vi "GetCurrentSnapshot.vi"(8 "error in (no error)":errorcluster, 11 "Logger in":refnum<class "Logger.lvclass">) -> (0 "error out":errorcluster, 2 "Snapshot":T1={"globalThreshold"=enum."INFO", "appenders"=[]}, 3 "Logger out":refnum<class "Logger.lvclass">)   [LabVIEW 2026, in "Lumberjack.lvlib" / "Logger.lvclass"]
doc: "Reads the logger's current published Snapshot without consuming it.\nNon-destructively reads the shared Snapshot notifier and returns globalThreshold plus the appenders array (RegistryEntry {id, enqueuer}) the manager last posted; reflects the state as of the last register/unregister/threshold change. Returns the empty/default Snapshot when no logger resolves.\nLumberjack.lvlib, Logger.lvclass, public."
uses:
  Logger.lvclass
  TypeDefs/Snapshot.ctl
  TypeDefs/Severity.ctl
  <vilib>/ActorFramework/Message Enqueuer/Message Enqueuer.lvclass
  Logger.lvclass/Logger.ctl
  Lumberjack.lvlib
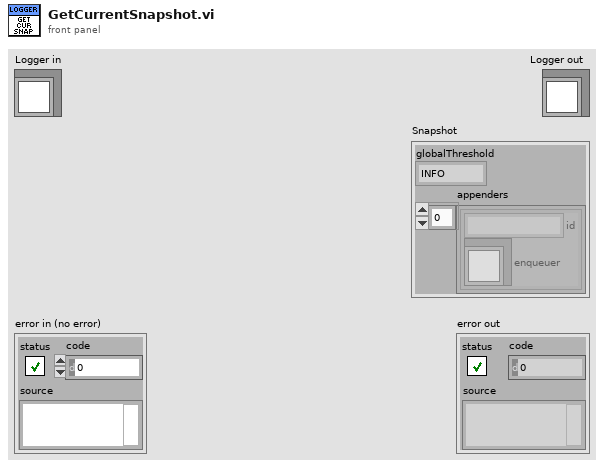
[diagram p1: front panel]
types:
  T1 = typedef "Lumberjack.lvlib/Snapshot.ctl" = cluster{"globalThreshold":T2, "appenders":cluster{"id":string, "enqueuer":refnum<class "Message Enqueuer.lvclass">}[]}
  T2 = typedef "Lumberjack.lvlib/Severity.ctl" = enum16{"OFF", "FATAL", "ERROR", "WARN", "INFO", "DEBUG", "TRACE", "ALL"}
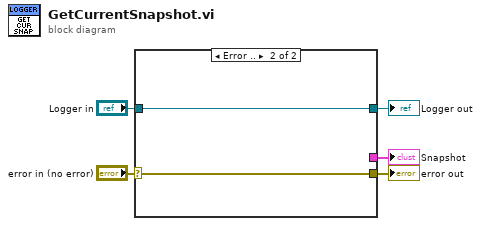
[diagram p0: block diagram]
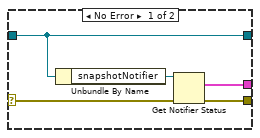
[diagram p2: hidden frame]
diagram:
  n1 = case shown="Error .." "error in (no error)" {
    selector: "error in (no error)" -> [w7 w12]
    tunnel: [w10 w12] -> w5
    tunnel: [w8 _] -> w4
    tunnel: "Logger in" -> [w6 w11]
    tunnel: [w6 w11] -> w1
    frame No Error {
      n2 = Unbundle By Name(w6) -> ("snapshotNotifier"=w9:refnum<notifier>)
      n3 = Get Notifier Status(notifier=w9, error in (no error)=w7) -> (current notification=w8:T1, error out=w10:errorcluster)  [unwired: 3 out]
    }
    frame Error {
    }
  }
  "error out" <- w5
  "Snapshot" <- w4
  "Logger out" <- w1
